vi "sort.vi"(2 "n":i32, 3 "Real":sgl[](array[numeric])=[0.0, 0.0, 0.0, 0.0, 0.0, 0.0, 0.0, 0.0, 0.0, 0.0, 0.0, 0.0, 0.0, 0.0, 0.0, 0.0, 0.0, 0.0, 0.0, 0.0]) -> (1 "Sorted A":sgl[](array[numeric]))   [LabVIEW 2020]
uses:
  <vilib>/rvi/Emulation/niFpgaGetClockAttributes.vi
  <vilib>/rvi/Emulation/niFpgaSctlEmulationGetInTimedLoop.vi
  <vilib>/rvi/Emulation/niFpgaEmulationReportErrorSimple.vi
  <vilib>/rvi/Emulation/niFpgaCriticalErrorInLSC.vi
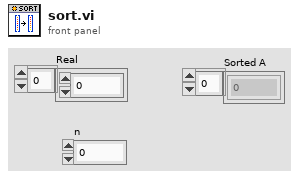
[diagram p1: front panel]
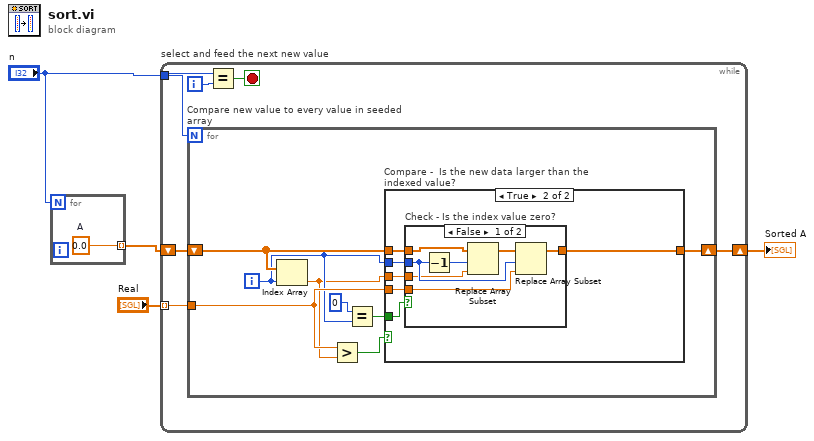
[diagram p0: block diagram]
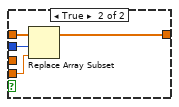
[diagram p3: hidden frame]
diagram:
  n1 = for {
    N: "n" -> [_]
    tunnel: [w5] -> w3 mode=indexing
    w5 = sgl 0.0  # A
  }
  n2 = while "select and feed the next new value" {
    shift-right: [w10] -> w4
    shift-left: w3 -> [w11]
    tunnel: "n" -> [w6]
    tunnel: "Real" -> [w7] mode=indexing
    i -> [w9]
    stop <- w8 stop-if-true
    n3 = for "Compare new value to every value in seeded array" {
      N: w6 -> [_]
      tunnel: w7 -> [w17]
      shift-right: [w16] -> w10
      shift-left: w11 -> [w18]
      i -> [w15]
      n4 = Index Array(array=w18, index=w15) -> (element=w12:sgl)
      n5 = Greater?(x=w17, y=w12) -> (0:w19:bool)
      n6 = Equal?(x=0, y=w15) -> (x = y?=w13:bool)
      n7 = case "Compare -  Is the new data larger than the indexed value?" shown="True" w19 {
        tunnel: w18 -> [w20 w25]
        tunnel: w13 -> [_ w26]
        tunnel: w17 -> [_ w24]
        tunnel: w15 -> [_ w23]
        tunnel: [w20 w22] -> w16
        tunnel: w12 -> [_ w21]
        frame False {
        }
        frame True {
          n8 = case "Check - Is the index value zero?" shown="False" w26 {
            tunnel: w25 -> [w29 w37]
            tunnel: w24 -> [w32 w36]
            tunnel: w23 -> [w28 w34]
            tunnel: [w31 w35] -> w22
            tunnel: w21 -> [w27 _]
            frame False {
              n9 = Decrement(x=w28) -> (x-1=w30:i32)
              n10 = Replace Array Subset(array=w29, new element=w27, index=w30) -> (w33:sgl[])
              n11 = Replace Array Subset(array=w33, new element=w32, index=w28) -> (w31:sgl[])
            }
            frame True {
              n12 = Replace Array Subset(array=w37, new element=w36, index=w34) -> (w35:sgl[])
            }
          }
        }
      }
    }
    n13 = Equal?(x=w6, y=w9) -> (x = y?=w8:bool)
  }
  "Sorted A" <- w4
